vi "Strip UTF8 Byte Order Mark (if present).vi"(11 "Text in":string) -> (2 "Mark was stripped":bool, 3 "Possible Byte Order Mark Stripped":string)   [LabVIEW 2020, in "JSONtext.lvlib"]
doc: "Removes any Byte Order Mark for UTF-8 that an external editor may have added."
uses:
  <vilib>/JDP Science/JSONtext/JSONtext.lvlib
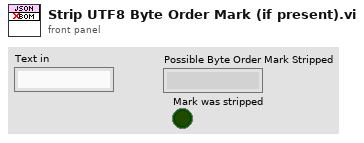
[diagram p1: front panel]
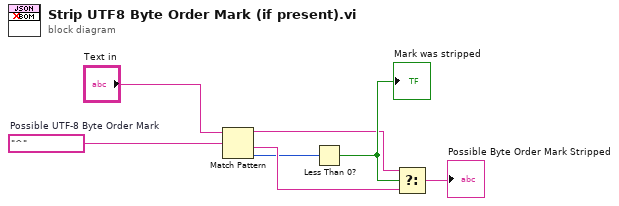
[diagram p0: block diagram]
diagram:
  w5 = "^﻿"  # Possible UTF-8 Byte Order Mark
  n1 = Match Pattern(string="Text in", regular expression=w5) -> (before substring=w2:string, after substring=w4:string, offset past match=w1:i32)  [unwired: 1 in, 1 out]
  n2 = Less Than 0?(x=w1) -> (x < 0?=w3:bool)
  "Mark was stripped" <- w3
  n3 = Select(t=w2, s=w3, f=w4) -> (s? t:f=→"Possible Byte Order Mark Stripped":string)
